vi "SetCommandValue.vi"(1 "error in (no error)":errorcluster, 2 "Feature Name":string, 3 "IGxDevice":refnum<k24>) -> (0 "error out":errorcluster)   [LabVIEW 2013, in "GxLVlib.lvlib"]
uses:
  GxLVlib.lvlib
  C:/Program Files/Daheng Imaging/GalaxySDK/Samples/LabVIEW SDK/x64/GxLVLib/dll/GxIAPINET.dll
  dll/GxIAPINET.dll
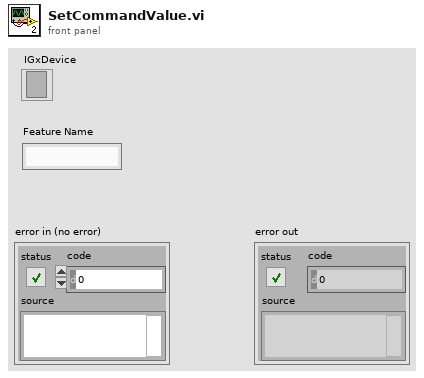
[diagram p1: front panel]
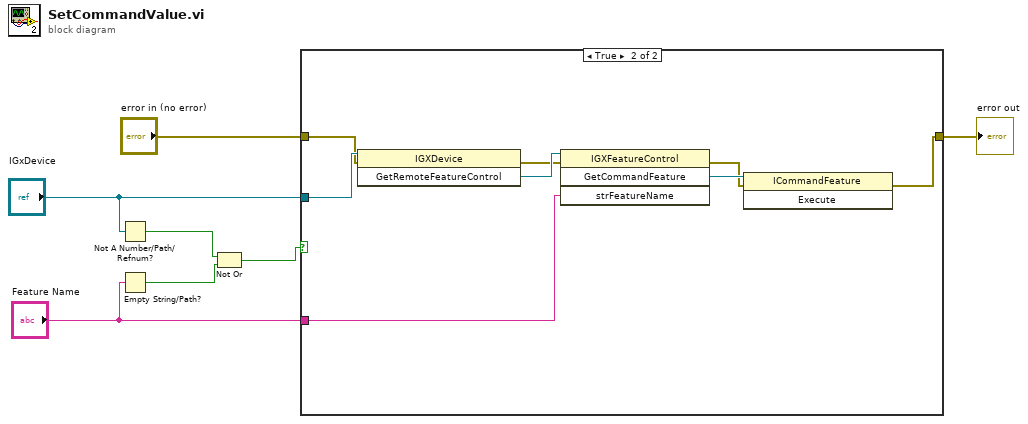
[diagram p0: block diagram]
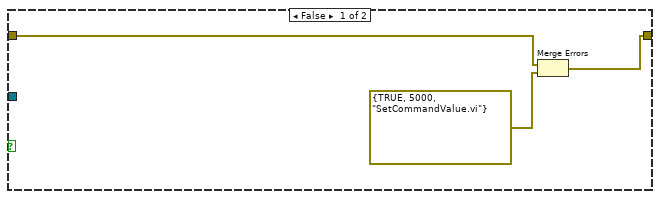
[diagram p2: hidden frame]
diagram:
  n1 = Not A Number/Path/Refnum?(number/path/refnum="IGxDevice") -> (NaN/Path/Refnum?=w7:bool)
  n2 = Empty String/Path?(string/path="Feature Name") -> (empty?=w6:bool)
  n3 = Not Or(1:w6, 2:w7) -> (0:w5:bool)
  n4 = case shown="True" w5 {
    tunnel: "error in (no error)" -> [w9 w17]
    tunnel: [w8 w11] -> w3
    tunnel: "IGxDevice" -> [_ w18]
    tunnel: "Feature Name" -> [_ w14]
    frame False {
      n5 = Merge Errors(w9, errorcluster {TRUE, 5000, "SetCommandValue.vi"}) -> (w8:errorcluster)
    }
    frame True {
      n6 = invoke class="IGXDevice" method="GetRemoteFeatureControl"(reference=w18, error in=w17) -> (error out=w15:errorcluster, "GetRemoteFeatureControl"=w16:refnum<k24>)  [unwired: 1 in, 1 out]
      n7 = invoke class="IGXFeatureControl" method="GetCommandFeature"(reference=w16, error in=w15, "strFeatureName"=w14) -> (error out=w12:errorcluster, "GetCommandFeature"=w13:refnum<k24>)  [unwired: 1 in, 2 out]
      n8 = invoke class="ICommandFeature" method="Execute"(reference=w13, error in=w12) -> (error out=w11:errorcluster)  [unwired: 1 in, 2 out]
    }
  }
  "error out" <- w3
